vi "Swerve Drive periodic.vi"(0 "X":dbl(slide) scale=-1.0..1.0, 7 "Y":dbl(slide) scale=1.0..-1.0, 11 "Z":dbl(knob) scale=1.0..-1.0, 12 "Auto Controls":bool, 13 "Field Centric":bool) -> ()   [LabVIEW 2016]
uses:
  <vilib>/Rock Robotics/WPI/ThirdParty/CanMotor/TalonSRX/WPI_CANTalonSRX_APIControlMode.ctl
  <vilib>/Rock Robotics/WPI/ThirdParty/CanMotor/TalonSRX/WPI_CANTalonSRX_APIFeedbackSelect.ctl
  VI-Database/Swerve Drive/4.0/Apple Gyro/Apple Pi Gyro Library.lvlib
panel:
  in  "Reverse Feedback Sensor":bool
  in  "Recalculate Distance":bool=TRUE
  in  "Rot. Point X":dbl
  in  "Rot. Point Y":dbl
  in  "Deadband":dbl=0.04 format="%#_13g"
  in  "Debug?":bool
  in  "Motor":bool[](array[boolean])=[FALSE, FALSE, FALSE, FALSE]
  in  "PIDF":cluster{"P":dbl, "I":dbl, "D":dbl, "F":dbl}
  in  "Robot Width":dbl=21.5
  in  "Robot Length":dbl=21.5
  in  "Reset Current":bool
  in  "Override NT?":bool
  in  "Gyro Select (Overide)":enum16{"IMU", "SPI", "Analog", "Navx"}(ring)
  # "FR"
  # "FL"
  # "BR"
  # "FL"
  # "SWERVE DRIVE\nVersion 1.0 periodic\nCory Lynch\nChris Garuti\nGavin Popkin\nApple Pi Robotics\nTeam 2067"
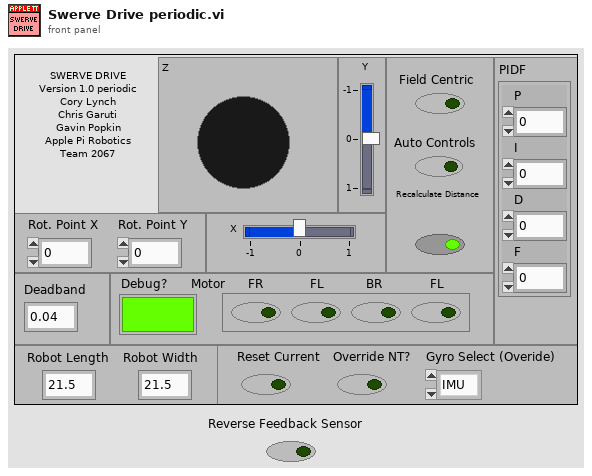
[diagram p1: front panel]
types:
  T1 = typedef "WPI_CANTalonSRX_APIControlMode.ctl" = enum8{"Percent VBus", "Speed", "Position", "Slave", "Unchanged / Invalid", "Voltage Compensation", "Current", "Motion Profile", "Motion Magic"}
  T2 = typedef "WPI_CANTalonSRX_GlobalStatus.ctl" = cluster{"Applied Throttle":dbl, "Module Enabled":bool, "CAN Error":errorcluster, "Closed Loop Error":dbl, "Forward Limit Switch Closed":bool, "Reverse Limit Switch Closed":bool, "Sensor Position":dbl, "Sensor Velocity":dbl, "Current":dbl, "Sticky Fault - Over Temp":bool, "Sticky Fault - Under Voltage":bool, "Sticky Fault - Forward Limit":bool, "Sticky Fault - Reverse Limit":bool, "Sticky Fault - Forward Soft Limit":bool, "Sticky Fault - Reverse Soft Limit":bool, "Brake is Enabled":bool, "Encoder Position":dbl, "Encoder Velocity":dbl, "Encoder Index Count":dbl, "Encoder A Pin State":bool, "Encoder B Pin State":bool, "Encoder Index Pin State":bool, "Analog In":dbl, "Analog In Velocity":dbl, "Temperature (C)":dbl, "Battery Voltage":dbl, "Control 5 Is Supported":bool, "Current Profile Slot Select":dbl, "Pos Div 8":bool, "Vel Div 4":bool, "Pulse Width Position":i32, "Pulse Width Velocity":i32, "Pulse Width Rise To Rise (us)":i32, "Pulse Width Rise To Fall (us)":i32, "Mot Prof Active Is Under Run":bool, "Mot Prof Active Has Under Run":bool, "Mot Prof Active Is Last":bool, "Mot Prof Active Velocity Only":bool, "Mot Prof Active Is Valid":bool, "Mot Prof Buffer Is Full":bool, "Mot Prof Active Profile Slot Select":i32, "Mot Prof NextID":i32, "Mot Prof Count":i32, "Mot Prof Active Velocity":dbl, "Mot Prof Active Position":dbl, "Mot Prof Output Enable":i32}
  T3 = typedef "WPI_CANTalonSRX_APIFeedbackSelect.ctl" = enum16{"Digital Quadrature Encoder", "Analog Potentiometer", "Analog Encoder", "Count on Quad-A (Rising-Edge)", "Count on Quad-A (Falling-Edge)", "CTR Magnetic Enc (Absolute)", "CTR Magnetic Enc (Relative)", "Pulse Width"}
  T4 = typedef "WPI_MotorControlDeviceRef.ctl" = cluster{"DeviceStatus":errorcluster, "Type":T5, "PWM":cluster{"PWM Channel":T6, "DeadBand":T7}, "CAN":cluster{"Device Number":u8, "SetOutput VI Ref":variant, "GetOutput VI Ref":variant, "Enable VI Ref":variant, "Disable VI Ref":variant, "Data":variant}, "Invert":bool}
  T5 = typedef "WPI_MotorControlType.ctl" = enum16{"PWM", "CAN"}
  T6 = typedef "FPGA_DIOPWMChannel.ctl" = enum8{"PWM 0", "PWM 1", "PWM 2", "PWM 3", "PWM 4", "PWM 5", "PWM 6", "PWM 7", "PWM 8", "PWM 9", "PWM MXP 0", "PWM MXP 1", "PWM MXP 2", "PWM MXP 3", "PWM MXP 4", "PWM MXP 5", "PWM MXP 6", "PWM MXP 7", "PWM MXP 8", "PWM MXP 9", "Invalid"}
  T7 = typedef "WPI_PWMDeadband.ctl" = cluster{"Name":string, "maxPositivePwm":i32, "minPositivePwm":i32, "centerPwm":i32, "maxNegativePwm":i32, "minNegativePwm":i32, "angularRange":u16}
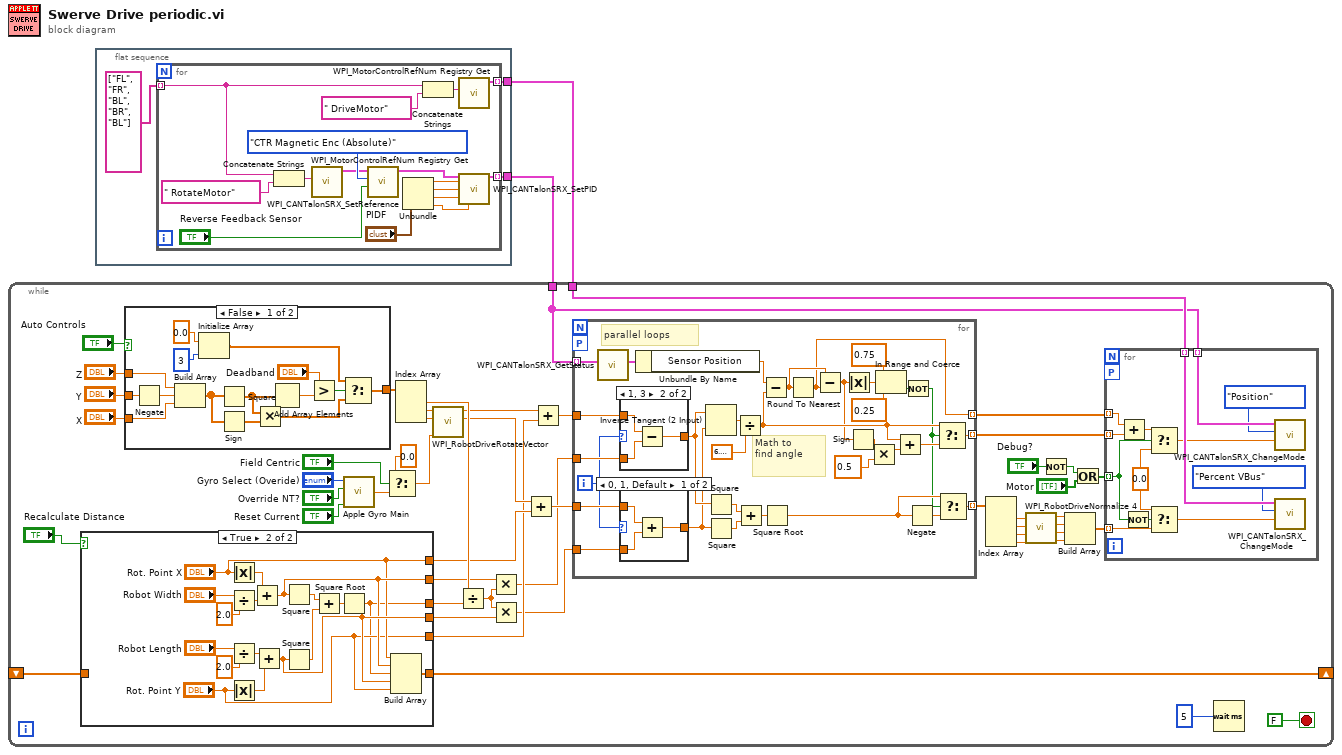
[diagram p0: block diagram]
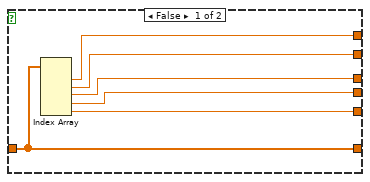
[diagram p2: hidden frame]
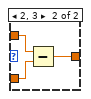
[diagram p3: hidden frame]
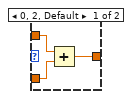
[diagram p4: hidden frame]
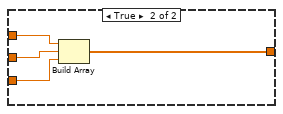
[diagram p5: hidden frame]
diagram:
  n1 = while {
    tunnel: w2 -> [w19]
    tunnel: w1 -> [w15]
    shift-right: [w24] -> _
    shift-left: _ -> [w23]
    stop <- FALSE stop-if-true
    n2 = case shown="True" "Recalculate Distance" {
      tunnel: [w70 w76] -> w30
      tunnel: [w67 "Rot. Point Y"] -> w26
      tunnel: [w71 "Rot. Point X"] -> w28
      tunnel: [w69 w72] -> w21
      tunnel: [w68 w77] -> w25
      tunnel: [w66 w73] -> w24
      tunnel: w23 -> [w66 _]
      frame False {
        n3 = Index Array(array=w66) -> (element #1=w71:dbl, element #2=w70:dbl, element #3=w69:dbl, element #4=w68:dbl, element #5=w67:dbl)  [unwired: 5 in]
      }
      frame True {
        n4 = Absolute Value(x="Rot. Point X") -> (abs(x)=w78:dbl)
        n5 = Divide(x="Robot Width", y=2.0) -> (x/y=w81:dbl)
        n6 = Divide(x="Robot Length", y=2.0) -> (x/y=w80:dbl)
        n7 = Absolute Value(x="Rot. Point Y") -> (abs(x)=w79:dbl)
        n8 = Add(x=w78, y=w81) -> (x+y=w76:dbl)
        n9 = Add(x=w80, y=w79) -> (x+y=w77:dbl)
        n10 = Square(x=w76) -> (x^2=w86:dbl)
        n11 = Square(x=w77) -> (x^2=w83:dbl)
        n12 = Add(x=w86, y=w83) -> (x+y=w87:dbl)
        n13 = Square Root(x=w87) -> (sqrt(x)=w72:dbl)
        n14 = Build Array("Rot. Point X", w76, w72, w77, "Rot. Point Y") -> (w73:dbl[])
      }
    }
    n15 = case shown="False" "Auto Controls" {
      tunnel: "Y" -> [w136 w150]
      tunnel: "X" -> [w141 w151]
      tunnel: "Z" -> [w138 w148]
      tunnel: [w139 w149] -> w49
      frame False {
        n16 = Negate(x=w136) -> (-x=w133:dbl)
        n17 = Build Array(w138, w133, w141) -> (w144:dbl[])
        n18 = Initialize Array(0.0 ("element"), 3 ("dimension size")) -> (w146:dbl[])
        n19 = Square(x=w144) -> (x^2=w142:dbl[])
        n20 = Sign(1:w144) -> (0:w143:dbl[])
        n21 = Multiply(x=w142, y=w143) -> (x*y=w140:dbl[])
        n22 = Add Array Elements(numeric array=w142) -> (sum=w135:dbl)
        n23 = Greater?(x="Deadband", y=w135) -> (0:w147:bool)
        n24 = Select(t=w146, s=w147, f=w140) -> (s? t:f=w139:dbl[])
      }
      frame True {
        n25 = Build Array(w148, w150, w151) -> (w149:dbl[])
      }
    }
    n26 = call "Apple Gyro Main.vi"("Reset Current"="Reset Current", "Override NT?"="Override NT?", "Gyro Select (Overide)"="Gyro Select (Overide)") -> ("Gyro Yaw Out"=w8:dbl)  [unwired: 1 in]
    n27 = Select(t=0.0, s="Field Centric", f=w8) -> (s? t:f=w22:dbl)
    n28 = Index Array(array=w49) -> (element #1=w47:dbl, element #2=w32:dbl, element #3=w31:dbl)  [unwired: 3 in]
    n29 = call <vilib>:"WPI_RobotDriveRotateVector.vi"("Angle"=w22, "X"=w31, "Y"=w32) -> ("X'"=w44:dbl, "Y'"=w43:dbl)  [unwired: 7 out]
    n30 = Divide(x=w47, y=w21) -> (x/y=w46:dbl)
    n31 = Multiply(x=w30, y=w46) -> (x*y=w11:dbl)
    n32 = Multiply(x=w46, y=w25) -> (x*y=w10:dbl)
    n33 = Add(x=w44, y=w28) -> (x+y=w29:dbl)
    n34 = Add(x=w43, y=w26) -> (x+y=w27:dbl)
    n35 = for {
      tunnel: w27 -> [w120]
      tunnel: w11 -> [w119]
      tunnel: w29 -> [w118]
      tunnel: w10 -> [w117]
      tunnel: [w110] -> w41 mode=indexing
      tunnel: [w103] -> w14 mode=indexing
      workers-P: _ -> [_]
      tunnel: w15 -> [w106] mode=indexing
      tunnel: [w90] -> w9 mode=indexing
      i -> [w116]
      # "parallel loops"
      # "Math to\nfind angle"
      n36 = call <vilib>:"WPI_CANTalonSRX_GetStatus.vi"("CAN Talon SRX Ref"=w106) -> ("Talon SRX Status"=w89:T2)  [unwired: 8 in, 2 out]
      n37 = case shown="1, 3" w116 {
        tunnel: w120 -> [w129 w132]
        tunnel: w119 -> [w128 w131]
        tunnel: [w127 w130] -> w105
        frame 0, 2, Default {
          n38 = Add(x=w129, y=w128) -> (x+y=w127:dbl)
        }
        frame 1, 3 {
          n39 = Subtract(x=w132, y=w131) -> (x-y=w130:dbl)
        }
      }
      n40 = case shown="0, 1, Default" w116 {
        tunnel: w118 -> [w123 w126]
        tunnel: w117 -> [w122 w125]
        tunnel: [w121 w124] -> w104
        frame 0, 1, Default {
          n41 = Add(x=w123, y=w122) -> (x+y=w121:dbl)
        }
        frame 2, 3 {
          n42 = Subtract(x=w126, y=w125) -> (x-y=w124:dbl)
        }
      }
      n43 = Unbundle By Name(w89) -> ("Sensor Position"=w96:dbl)
      n44 = Inverse Tangent (2 Input)(1:w104, 2:w105) -> (0:w108:dbl)
      n45 = Square(x=w105) -> (x^2=w114:dbl)
      n46 = Square(x=w104) -> (x^2=w115:dbl)
      n47 = Divide(x=w108, y=6.283185307179586) -> (x/y=w100:dbl)
      n48 = Add(x=w114, y=w115) -> (x+y=w113:dbl)
      n49 = Subtract(x=w96, y=w100) -> (x-y=w94:dbl)
      n50 = Square Root(x=w113) -> (sqrt(x)=w111:dbl)
      n51 = Round To Nearest(number=w94) -> (nearest integer value=w90:dbl)
      n52 = Subtract(x=w94, y=w90) -> (x-y=w95:dbl)
      n53 = Absolute Value(x=w95) -> (abs(x)=w98:dbl)
      n54 = Sign(1:w95) -> (0:w99:dbl)
      n55 = Multiply(x=w99, y=0.5) -> (x*y=w101:dbl)
      n56 = In Range and Coerce(upper limit=0.75, x=w98, lower limit=0.25) -> (In Range?=w93:bool)  [unwired: 1 out]
      n57 = Add(x=w100, y=w101) -> (x+y=w107:dbl)
      n58 = Not(x=w93) -> (.not. x?=w92:bool)
      n59 = Negate(x=w111) -> (-x=w112:dbl)
      n60 = Select(t=w100, s=w92, f=w107) -> (s? t:f=w103:dbl)
      n61 = Select(t=w111, s=w92, f=w112) -> (s? t:f=w110:dbl)
    }
    n62 = Index Array(array=w41) -> (element #1=w40:dbl, element #2=w39:dbl, element #3=w38:dbl, element #4=w37:dbl)  [unwired: 4 in]
    n63 = call <vilib>:"WPI_RobotDriveNormalize 4.vi"("D"=w37, "C"=w38, "B"=w39, "A"=w40) -> ("D'"=w33:dbl, "C'"=w34:dbl, "B'"=w35:dbl, "A'"=w36:dbl)
    n64 = Not(x="Debug?") -> (.not. x?=w12:bool)
    n65 = Build Array(w36, w35, w34, w33) -> (w13:dbl[])
    n66 = Or(x=w12, y="Motor") -> (x .or. y?=w18:bool[])
    n67 = for {
      tunnel: w14 -> [w60] mode=indexing
      tunnel: w15 -> [w65] mode=indexing
      tunnel: w13 -> [w61] mode=indexing
      tunnel: w19 -> [w64] mode=indexing
      tunnel: w18 -> [w59] mode=indexing
      workers-P: _ -> [_]
      tunnel: w9 -> [w56] mode=indexing
      w58 = 0.0
      n68 = Add(x=w56, y=w60) -> (x+y=w55:dbl)
      n69 = Not(x=w59) -> (.not. x?=w62:bool)
      n70 = Select(t=w55, s=w59, f=w58) -> (s? t:f=w57:dbl)
      n71 = Select(t=w58, s=w62, f=w61) -> (s? t:f=w63:dbl)
      n72 = call <vilib>:"WPI_CANTalonSRX_ChangeMode.vi"("Output"=w57, "Control Mode"=WPI_CANTalonSRX_APIControlMode."Position", "CAN Talon SRX Ref"=w65) -> ()  [unwired: 7 in, 2 out]
      n73 = call <vilib>:"WPI_CANTalonSRX_ChangeMode.vi"("Output"=w63, "Control Mode"=WPI_CANTalonSRX_APIControlMode."Percent VBus", "CAN Talon SRX Ref"=w64) -> ()  [unwired: 7 in, 2 out]
    }
    n74 = Wait (ms)(milliseconds to wait=u32 5) -> ()  [unwired: 1 out]
  }
  n75 = flat-sequence {
    tunnel: [w153] -> w2
    tunnel: [w152] -> w1
    frame #0 {
      n76 = for {
        tunnel: string[] ["FL", "FR", "BL", "BR", "BL"] -> [w164] mode=indexing
        tunnel: [w161] -> w153 mode=indexing
        tunnel: [w157] -> w152 mode=indexing
        n77 = Concatenate Strings(w164, " RotateMotor" ("refnum name")) -> (w163:string)
        n78 = call <vilib>:"WPI_MotorControlRefNum Registry Get.vi"("refnum name"=w163) -> ("MotorControlDevRef"=w165:T4)  [unwired: 9 in, 1 out]
        n79 = call <vilib>:"WPI_CANTalonSRX_SetReference.vi"("Reverse Feedback Sensor"="Reverse Feedback Sensor", "Feedback Reference"=WPI_CANTalonSRX_APIFeedbackSelect."CTR Magnetic Enc (Absolute)", "CAN Talon SRX Ref"=w165) -> ("CAN Talon SRX Ref"=w159:T4)  [unwired: 7 in, 1 out]
        n80 = Unbundle("PIDF") -> ("P"=w166:dbl, "I"=w168:dbl, "D"=w167:dbl, "F"=w156:dbl)
        n81 = Concatenate Strings(w164, " DriveMotor") -> (w162:string)
        n82 = call <vilib>:"WPI_MotorControlRefNum Registry Get.vi"("refnum name"=w162) -> ("MotorControlDevRef"=w161:T4)  [unwired: 9 in, 1 out]
        n83 = call <vilib>:"WPI_CANTalonSRX_SetPID.vi"("CAN Talon SRX Ref"=w159, "P"=w166, "I"=w168, "D"=w167, "F"=w156) -> ("CAN Talon SRX Ref"=w157:T4)  [unwired: 9 in, 1 out]
      }
    }
  }
